vi "Set Room Lamp State.vi"(8 "error in (no error)":errorcluster, 9 "Value":bool, 10 "Room List":T1, 11 "Light Control in":refnum<class "Light Control.lvclass">) -> (0 "error out":errorcluster, 3 "Light Control out":refnum<class "Light Control.lvclass">)   [LabVIEW 2021, in "Light Control.lvlib" / "Light Control.lvclass"]
uses:
  Light Control.lvclass
  Room List.ctl
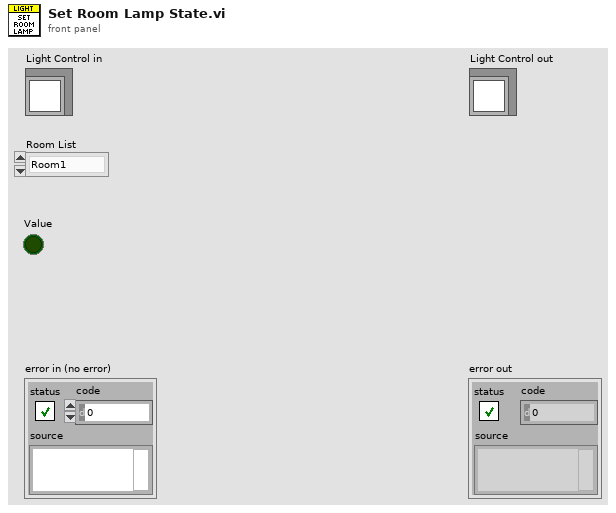
[diagram p1: front panel]
types:
  T1 = typedef "Light Control.lvlib/Light Control.lvclass/Room List.ctl" = enum16{"Room1", "Room2"}
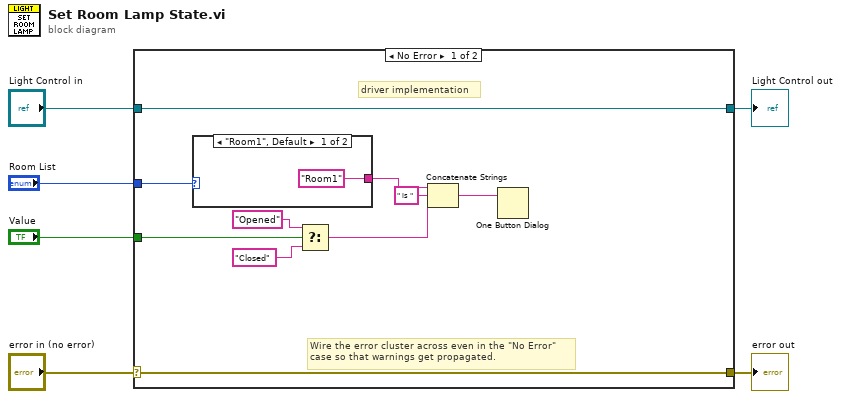
[diagram p0: block diagram]
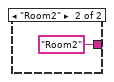
[diagram p2: hidden frame]
diagram:
  n1 = case shown="No Error" "error in (no error)" {
    selector: "error in (no error)" -> [w15 w20]
    tunnel: [w15 w20] -> w5
    tunnel: [w16 w19] -> w3
    tunnel: "Light Control in" -> [w16 w19]
    tunnel: "Room List" -> [w14 _]
    tunnel: "Value" -> [w13 _]
    frame No Error {
      # "driver implementation"
      # "Wire the error cluster across even in the \"No Error\"\ncase so that warnings get propagated."
      n2 = case shown="\"Room1\", Default" w14 {
        tunnel: ["Room1" "Room2"] -> w10
        frame "Room1", Default {
        }
        frame "Room2" {
        }
      }
      n3 = Select(t="Opened", s=w13, f="Closed") -> (s? t:f=w8:string)
      n4 = Concatenate Strings(w10, " is " ("string"), w8) -> (w7:string)
      n5 = One Button Dialog(message=w7) -> ()  [unwired: 1 in, 1 out]
    }
    frame Error {
    }
  }
  "error out" <- w5
  "Light Control out" <- w3
